vi "onProcessStarted.vi"(8 "error in (no error)":errorcluster, 11 "Microscope":refnum<class "Microscope.lvclass">) -> (0 "error out":errorcluster, 3 "Microscope out":refnum<class "Microscope.lvclass">)   [LabVIEW 2013, in "Microscope.lvclass"]
doc: "JKI State Machine Objects (SMO) 1.0.4.18\nJKI - JKI\nCopyright (c) 2016, JKI"
uses:
  Microscope.lvclass
  <vilib>/JKI/JKI SMO/SMO/SMO.lvclass
panel:
  # "For instructions on how to use the JKI State Machine Objects, examples and video tutorials, visit:\nhttp://jki.net/state-machine-objects/\n\nJKI State Machine Objects™\nhttp://jki.net/state-machine-objects/\nCopyright (C) 2005-2015, JKI <info@jki.net>\nALL RIGHTS RESERVED"
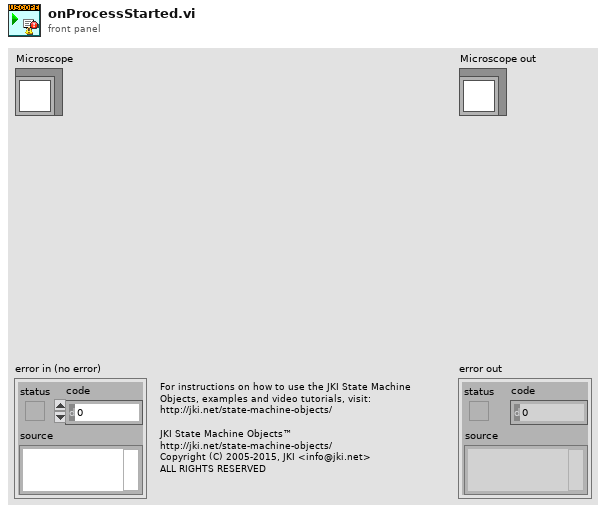
[diagram p1: front panel]
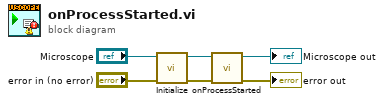
[diagram p0: block diagram]
diagram:
  n1 = call "Initialize.vi"("error in (no error)"="error in (no error)", "Microscope"="Microscope") -> ("error out"=w1:errorcluster, "Microscope out"=w3:refnum<class "Microscope.lvclass">)  [unwired: 8 in]
  n2 = call-parent "onProcessStarted.vi"("error in (no error)"=w1, "SMO"=w3) -> ("error out"=→"error out":errorcluster, "SMO out"=→"Microscope out":refnum<class "Microscope.lvclass">)  [unwired: 8 in]
